vi "DAQNavi Write (Buffered Counter Pulse Width).vi"(7 "data":cluster{"high period":dbl, "low period":dbl}[][](array[cluster]), 8 "error in (no error)":errorcluster, 9 "number of samples per channel to write":i32=10, 10 "timeout":dbl=10.0, 11 "task in":i32) -> (0 "error out":errorcluster, 3 "task out":i32)   [LabVIEW 2020]
uses:
  DAQNavi_LV.dll
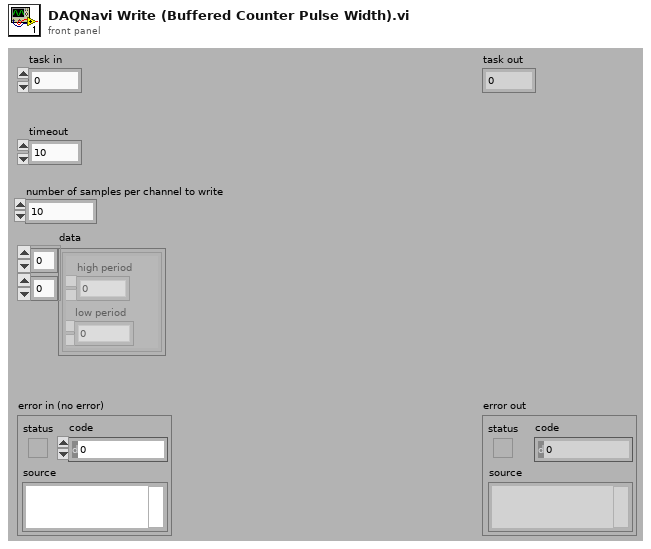
[diagram p1: front panel]
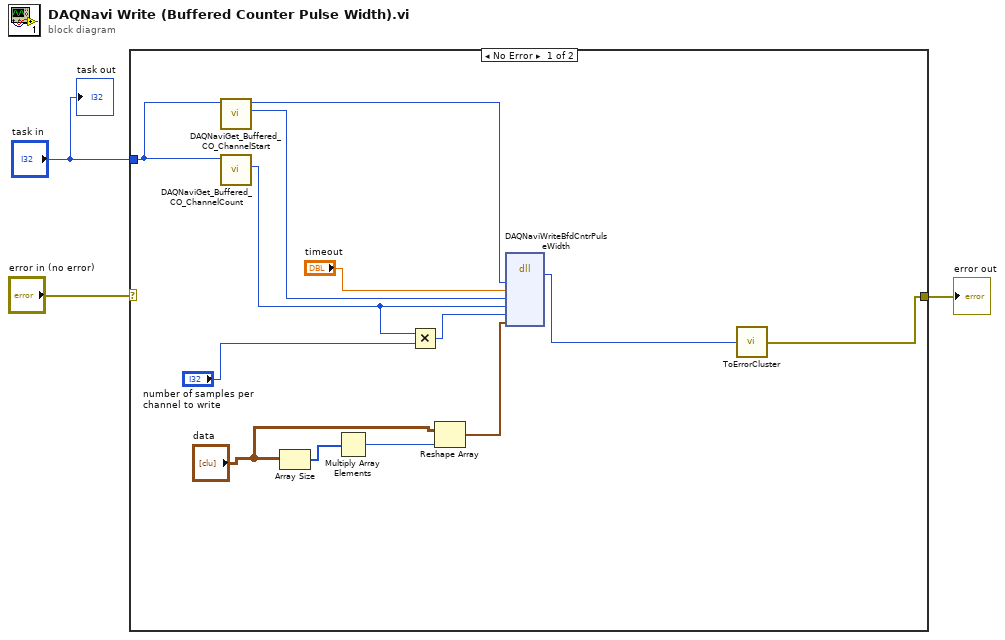
[diagram p0: block diagram]
diagram:
  n1 = case shown="No Error" "error in (no error)" {
    selector: "error in (no error)" -> [_ w17]
    tunnel: [w4 w17] -> w2
    tunnel: "task in" -> [w16 _]
    frame No Error {
      n2 = call "DAQNaviGet_Buffered_CO_ChannelStart.vi"("task in"=w16) -> ("channelStart"=w15:i32, "task out"=w13:i32)  [unwired: 1 in, 8 out]
      n3 = call "DAQNaviGet_Buffered_CO_ChannelCount.vi"("task in"=w16) -> ("channelCount"=w7:i32)  [unwired: 1 in, 9 out]
      n4 = Array Size(array="data") -> (size(s)=w12:i32[])
      n5 = Multiply Array Elements(1:w12) -> (0:w11:i32)
      n6 = Multiply(x=w7, y="number of samples per channel to write") -> (x*y=w6:i32)
      n7 = Reshape Array("data", w11) -> (w9:cluster{"high period":dbl, "low period":dbl}[])
      n8 = dll-call lib="DAQNavi_LV.dll" fn="DAQNaviWriteBfdCntrPulseWidth"("taskID"=w13, "timeout"="timeout", "cntrStart"=w15, "cntrCount"=w7, "count"=w6, "samples"=w9) -> ("return type"=w5:i32)  [unwired: 9 in, 2 out]
      n9 = call "ToErrorCluster.vi"("error code"=w5) -> ("error out"=w4:errorcluster)
    }
    frame Error {
    }
  }
  "error out" <- w2
  "task out" <- "task in"
